vi "EventLog.File.ReadWrite.vi"(6 "read count (ALL)":i32=-1, 7 "action (read)":enum16{"read", "write", "get size"}(ring), 8 "error in":errorcluster, 9 "read offset [records]":i64, 10 "event in":T1={"ts"=0.0, "lev"=enum."Debug", "src"=enum."All", "msg"=enum."Log out", "arg"=[]} {"ts" format="%<%X\n%x>T"}, 11 "file":path) -> (0 "error out":errorcluster, 1 "offset [B]":i64, 2 "Events out":T5[](array[typedef]) {"ts" format="%<%X\n%x>T"}, 3 "size [B]":i64, 4 "End of File?":bool)   [LabVIEW 2016]
uses:
  EventLog.EventGui.ctl
  EventLog.EventLevel.ctl
  EventLog.EventSource.ctl
  Translator/Translator.Message.ctl
  EventLog.Event.ctl
panel:
  out "size(s)":i32
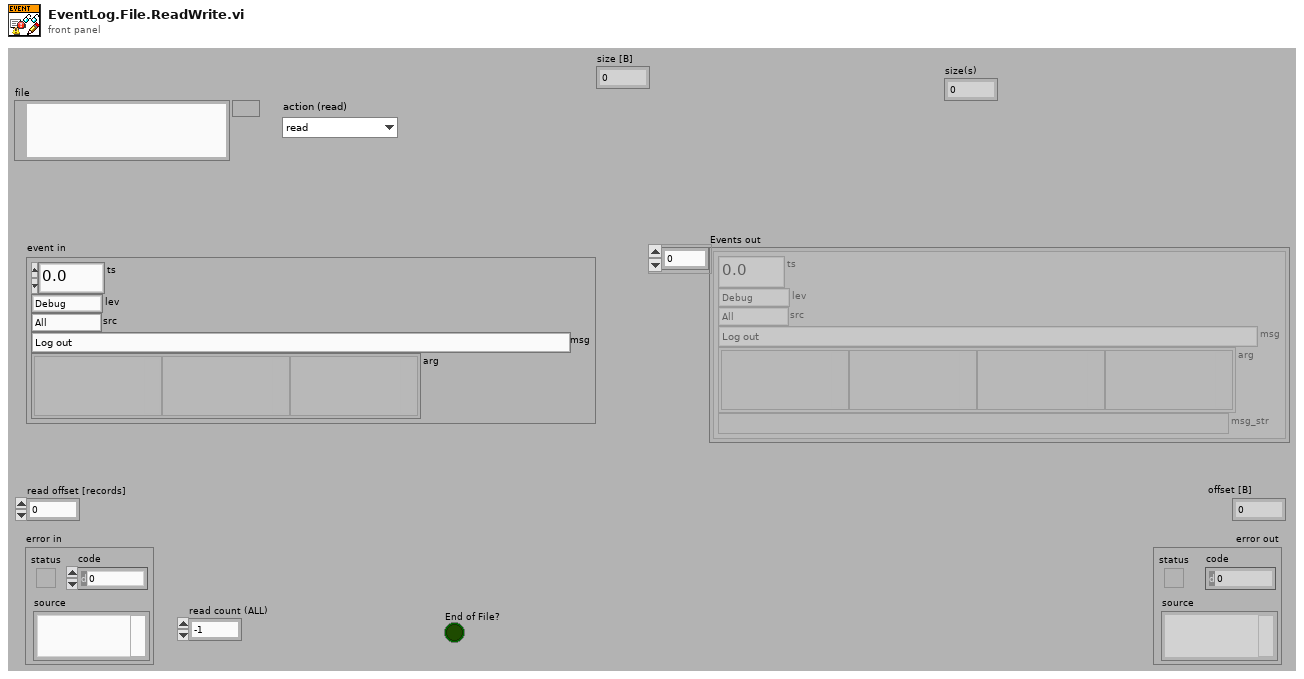
[diagram p1: front panel]
types:
  T1 = typedef "EventLog.Event.ctl" = cluster{"ts":dbl, "lev":T2, "src":T3, "msg":T4, "arg":variant[]}
  T2 = typedef "EventLog.EventLevel.ctl" = enum8{"Debug", "Info", "Warning", "Error"}
  T3 = typedef "EventLog.EventSource.ctl" = enum16{"All", "Gui", "Cache", "PLC1", "PLC2", "PLC3", "DB", "DB01", "DB02", "DB03", "DB04", "DB05", "DB06", "DB07", "DB08", "DB09", "DB10", "DB11", "DB12", "DB13", "DB14", "DB15", "DB16"}
  T4 = typedef "Translator.Message.ctl" = enum16{"-", "Event confirmed", "Log out", "Log in", "Shutdown", "Cancel", "Start", "Continue", "Stop", "On", "Off", "OK", "NOK", "NOK %s", "This", "Prev", "Home", "Work", "In progress...", "Missing", "Empty", "Hardware failure", "Initial", "Error %d >> %s", "Error %d >> %s >> %s", "Starting %s", "Quitting %s", "Configured", "Initializing", "Quitting", "Loading", "Running %s", "Stopped", "Summary", "Do you want to continue?", "Do you want to exit?", "Log out?", "System", "All", "IDLE", "Translating...%s", "Not found", "Alarm %s", "Run", "Skip", "Abort", "Repeat", "Please wait...", "Database disconnected", "Login to database successful", "Login to database failed: %d; %s", "Get process step data for %s", "Changeover off", "Changeover into %s", "Product %s | %s found in cache with status %d at previous station", "Product %s | %s found in database with status %d at previous station", "Product %s | %s not found in cache at previous station", "Product %s | %s not found in database at previous station", "Product %s | %s found in cache with status %d at this station (%d repetion)", "Product %s | %s found in database with status %d at this station (%d repetition)", "Product %s | %s not found in cache at this station", "Product %s | %s not found in database at this station", "Product %s | %s found in cache for component %s | %s", "Product %s | %s found in database for component %s | %s", "Product not found in cache for component %s | %s", "Product not found in database for component %s | %s", "Product %s | %s connected with component %s | %s (cache)", "Product %s | %s connected with component %s | %s (database)", "New data for %s | %s (cache)", "New data for %s | %s (database)", "File %s moved (cache)", "File %s deleted (cache)", "Msg %d >> %s", "PLC LifeBit Failure", "Reconnecting DB", "Reconnecting PLC", "Free disk space is below 1GB - contact technician"}
  T5 = typedef "EventLog.EventGui.ctl" = cluster{"ts":dbl, "lev":T2, "src":T3, "msg":T4, "arg":variant[], "msg_str":string}
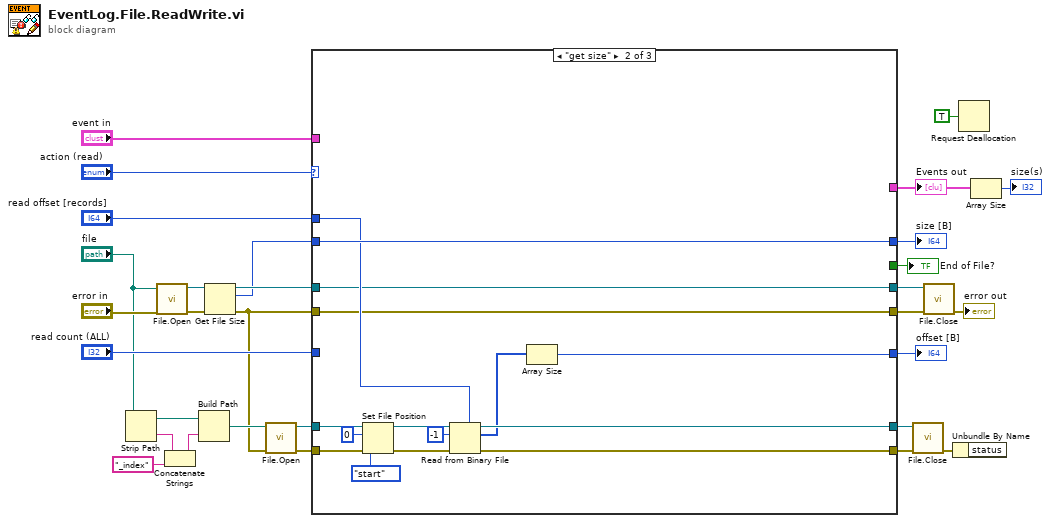
[diagram p0: block diagram]
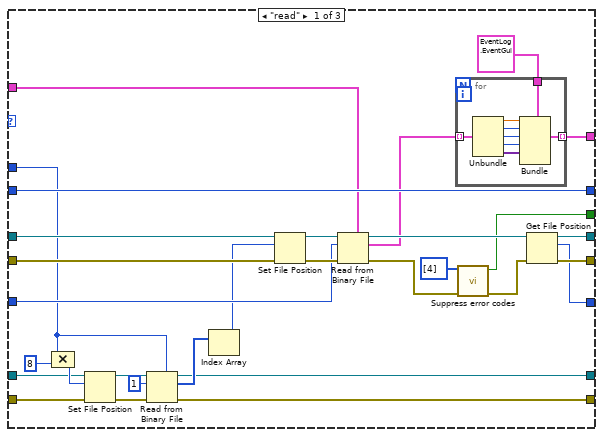
[diagram p2: hidden frame]
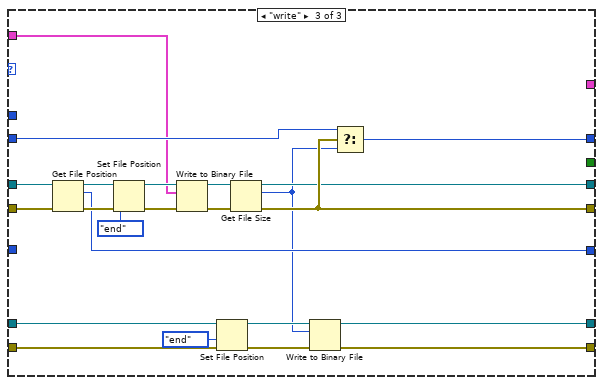
[diagram p3: hidden frame]
diagram:
  n1 = Strip Path(path="file") -> (stripped path=w12:path, name=w10:string)
  n2 = call "File.Open.vi"("error in"="error in", "file"="file") -> ("error out"=w18:errorcluster, "File ref out"=w17:refnum<file>)  [unwired: 8 in]
  n3 = Concatenate Strings(w10, "_index" ("string")) -> (w9:string)
  n4 = Build Path(base path=w12, name or relative path=w9) -> (appended path=w8:path)
  n5 = Get File Size(file=w17, error in=w18) -> (refnum out=w16:refnum<file>, size (in bytes)=w2:i64, 0:w1:errorcluster)
  n6 = call "File.Open.vi"("error in"=w1, "file"=w8) -> ("error out"=w7:errorcluster, "File ref out"=w6:refnum<file>)  [unwired: 8 in]
  n7 = case shown="\"get size\"" "action (read)" {
    tunnel: w16 -> [w49 w70 w94]
    tunnel: [w56 w70 w99] -> w22
    tunnel: [w55 w71 w100] -> w21
    tunnel: w1 -> [w50 w71 w93]
    tunnel: "event in" -> [w46 _ w92]
    tunnel: "read offset [records]" -> [w32 w75 _]
    tunnel: [w58 _ _] -> w25
    tunnel: "read count (ALL)" -> [w47 _ _]
    tunnel: [w54 w69 w101] -> w26
    tunnel: [w48 w83 w98] -> w23
    tunnel: [w51 _ _] -> w19
    tunnel: w2 -> [w48 w83 w95]
    tunnel: w7 -> [w39 w81 w89]
    tunnel: w6 -> [w40 w82 w91]
    tunnel: [w34 w77 w87] -> w5
    tunnel: [w33 w76 w86] -> w4
    frame "read" {
      n8 = Compound Arithmetic op=MULTIPLY(w32, i64 8) -> (w41:i64)
      n9 = Set File Position(offset (in bytes) (0)=w41, refnum=w40, error in=w39) -> (refnum out=w38:refnum<file>, error out=w37:errorcluster)  [unwired: 1 in]
      n10 = Read from Binary File(5:w32, 8:w37, 10:1 ("count (1)"), 11:w38) -> (0:w33:errorcluster, 2:w35:i64[], 3:w34:refnum<file>)  [unwired: 2 in, 1 out]
      n11 = Index Array(array=w35) -> (element=w31:i64)  [unwired: 1 in]
      n12 = Set File Position(offset (in bytes) (0)=w31, refnum=w49, error in=w50) -> (refnum out=w59:refnum<file>, error out=w60:errorcluster)  [unwired: 1 in]
      n13 = Read from Binary File(5:w46, 8:w60, 10:w47, 11:w59) -> (0:w45:errorcluster, 2:w44:T1[], 3:w57:refnum<file>)  [unwired: 2 in, 1 out]
      n14 = for {
        tunnel: w44 -> [w68] mode=indexing
        tunnel: T5 {"ts"=0.0, "lev"=enum."Debug", "src"=enum."All", "msg"=enum."Log out", "arg"=[], "msg_str"=""} ("event in") -> [w67]
        tunnel: [w64] -> w58 mode=indexing
        n15 = Unbundle(w68) -> ("ts"=w66:dbl, "lev"=w65:T2, "src"=w63:T3, "msg"=w62:T4, "arg"=w61:variant[])
        n16 = Bundle(cluster=w67, "ts"=w66, "lev"=w65, "src"=w63, "msg"=w62, "arg"=w61) -> (w64:T5)  [unwired: 1 in]
      }
      n17 = call "Suppress error codes.vi"("error in (no error)"=w45, "suppress codes([43])"=i32[] [4]) -> ("error out"=w52:errorcluster, "suppressed"=w51:bool)  [unwired: 8 in]
      n18 = Get File Position(4:w52, 7:w57) -> (0:w55:errorcluster, 2:w54:i64, 3:w56:refnum<file>)
    }
    frame "get size" {
      n19 = Set File Position(offset (in bytes) (0)=i64 0, refnum=w82, from (0:start)=enum16{"start", "end", "current"}."start", error in=w81) -> (refnum out=w80:refnum<file>, error out=w79:errorcluster)
      n20 = Read from Binary File(5:w75, 8:w79, 10:-1 ("count (1)"), 11:w80) -> (0:w76:errorcluster, 2:w72:i64[], 3:w77:refnum<file>)  [unwired: 2 in, 1 out]
      n21 = Array Size(array=w72) -> (size(s)=w69:i32)
    }
    frame "write" {
      n22 = Get File Position(4:w93, 7:w94) -> (0:w103:errorcluster, 2:w101:i64, 3:w102:refnum<file>)
      n23 = Set File Position(refnum=w102, from (0:start)=enum16{"start", "end", "current"}."end", error in=w103) -> (refnum out=w106:refnum<file>, error out=w105:errorcluster)  [unwired: 1 out]
      n24 = Write to Binary File(file (use dialog)=w106, data=w92, error in=w105) -> (refnum out=w97:refnum<file>, error out=w96:errorcluster)  [unwired: 3 in, 1 out]
      n25 = Set File Position(refnum=w91, from (0:start)=enum16{"start", "end", "current"}."end", error in=w89) -> (refnum out=w88:refnum<file>, error out=w85:errorcluster)  [unwired: 1 out]
      n26 = Get File Size(file=w97, error in=w96) -> (refnum out=w99:refnum<file>, size (in bytes)=w84:i64, 0:w100:errorcluster)
      n27 = Write to Binary File(file (use dialog)=w88, data=w84, error in=w85) -> (refnum out=w87:refnum<file>, error out=w86:errorcluster)  [unwired: 3 in, 1 out]
      n28 = Select(t=w95, s=w100, f=w84) -> (s? t:f=w98:i64)
    }
  }
  "Events out" <- w25
  "offset [B]" <- w26
  "size [B]" <- w23
  "End of File?" <- w19
  n29 = call "File.Close.vi"("error in"=w4, "File ref in"=w5) -> ("error out"=w3:errorcluster)  [unwired: 9 in]
  n30 = call "File.Close.vi"("error in"=w21, "File ref in"=w22) -> ("error out"=→"error out":errorcluster)  [unwired: 9 in]
  n31 = Unbundle By Name(w3) -> ()  [unwired: 1 out]
  n32 = Request Deallocation(TRUE ("flag")) -> ()
  n33 = Array Size(array=w25) -> (size(s)=→"size(s)":i32)
